vi "client.vi"() -> ()   [LabVIEW 2012]
panel:
  out "数据输出":string
  out "错误输出":errorcluster
  in  "读取的字节":i32
  in  "数据输入":string
  in  "远程端口或服务名称":u16
  in  "地址":string
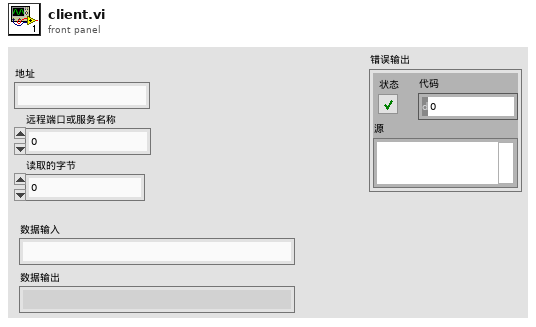
[diagram p1: front panel]
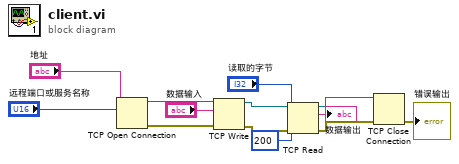
[diagram p0: block diagram]
diagram:
  n1 = TCP Open Connection(address="地址", remote port or service name="远程端口或服务名称") -> (connection ID=w11:refnum<k5>, error out=w10:errorcluster)  [unwired: 3 in]
  n2 = TCP Write(connection ID=w11, data in="数据输入", error in (no error)=w10) -> (connection ID out=w8:refnum<k5>, error out=w7:errorcluster)  [unwired: 1 in, 1 out]
  n3 = TCP Read(connection ID=w8, bytes to read="读取的字节", error in (no error)=w7, 9:200 ("超时毫秒(25000)")) -> (connection ID out=w4:refnum<k5>, data out=→"数据输出":string, error out=w3:errorcluster)  [unwired: 1 in]
  n4 = TCP Close Connection(connection ID=w4, error in (no error)=w3) -> (error out=→"错误输出":errorcluster)  [unwired: 1 in, 1 out]
